vi "Emballage_BDD_codeBarre_bdd.vi"(8 "Error in":errorcluster caption="Error in (no error)") -> (0 "Error out":errorcluster, 3 "tableau ajouté":string[][](array[string]))   [LabVIEW 2020]
uses:
  Modules/FS/60_FS_Controles/60_FS_SetGet.ctl
panel:
  out "tableau_code barre (article)":string[](array[string])
  out "tableau_Produit Code FAS (article)":string[](array[string])
  out "tableau_code barre":string[](array[string])
  out "tableau_Produit Code FAS":string[](array[string])
  out "Result Set":string[][](table) caption="Result Set (from first statement with results)"
  out "Column Names":string[](array[string])
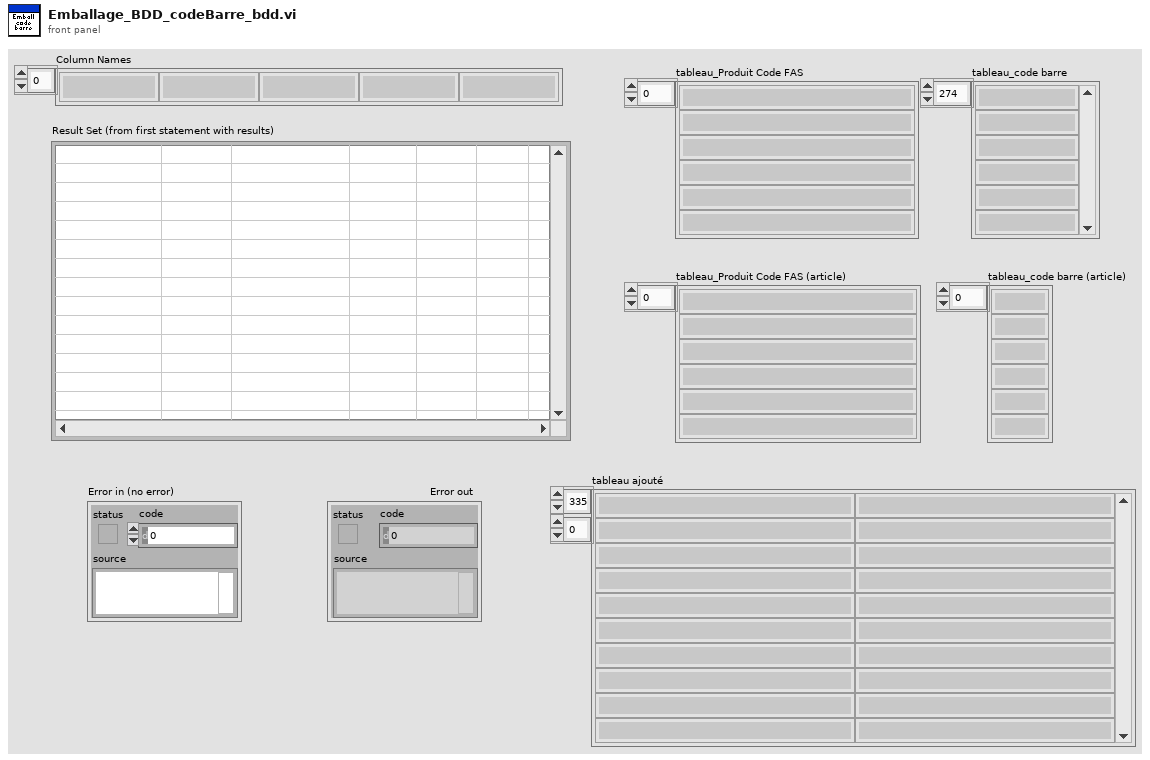
[diagram p1: front panel]
types:
  T1 = typedef "60_FS_SetGet.ctl" = enum16{"set", "get"}
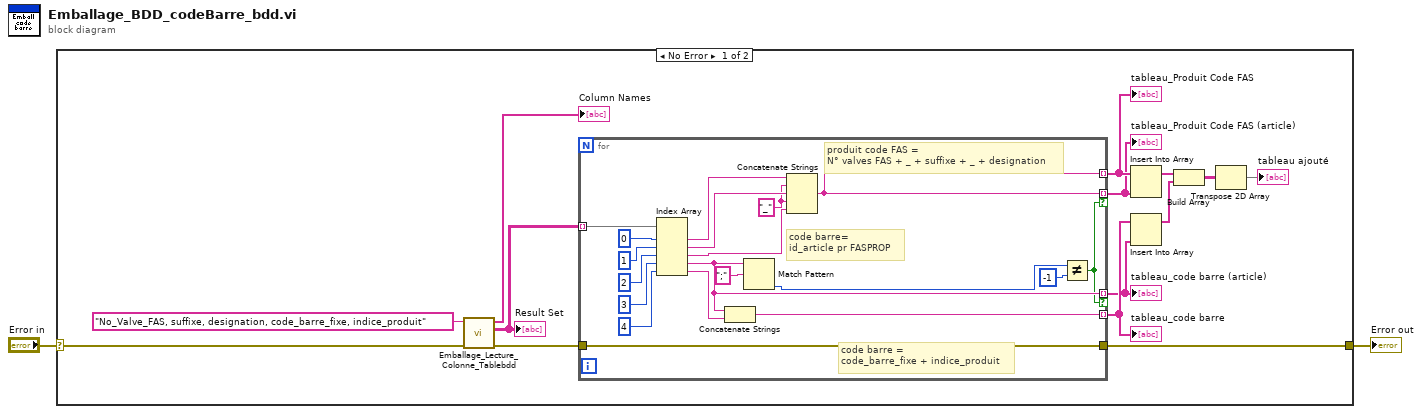
[diagram p0: block diagram]
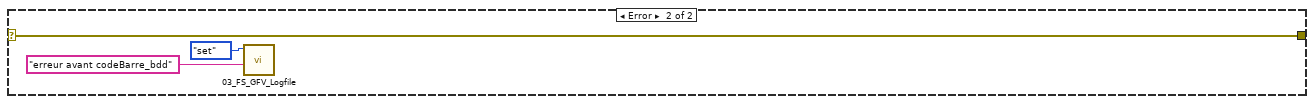
[diagram p2: hidden frame]
diagram:
  n1 = case shown="No Error" "Error in" {
    selector: "Error in" -> [w12 w38]
    tunnel: [w11 w38] -> w1
    frame No Error {
      n2 = call "Emballage_Lecture_Colonne_Tablebdd.vi"("Error in"=w12, "Colonne"="No_Valve_FAS, suffixe, designation, code_barre_fixe, indice_produit") -> ("Error out"=w13:errorcluster, "Result Set"=w14:string[][], "Column Names"=→"Column Names":string[])  [unwired: 6 in, 1 out]
      "Result Set" <- w14
      n3 = for {
        tunnel: w14 -> [w35] mode=indexing
        tunnel: [w19] -> w6 mode=indexing
        tunnel: [w24] -> w4 mode=indexing
        tunnel: w13 -> [w23]
        tunnel: [w23] -> w11
        tunnel: [w19] -> w5 mode=indexing if=w17
        tunnel: [w18] -> w3 mode=indexing if=w17
        w29 = "_" ("chaîne")
        # "code barre=\nid_article pr FASPROP"
        # "code barre =\ncode_barre_fixe + indice_produit"
        # "produit code FAS =\nN° valves FAS + _ + suffixe + _ + designation"
        n4 = Index Array(array=w35, index #1=0 ("indice"), index #2=1 ("indice"), index #3=2 ("indice"), index #4=3 ("indice"), index #5=4 ("indice")) -> (element #1=w31:string, element #2=w30:string, element #3=w28:string, element #4=w18:string, element #5=w25:string)
        n5 = Concatenate Strings(w18, w25) -> (w24:string)
        n6 = Match Pattern(string=w18, regular expression=";" ("expression régulière")) -> (offset past match=w21:i32)  [unwired: 1 in, 3 out]
        n7 = Concatenate Strings(w31, w29, w30, w29, w28) -> (w19:string)
        n8 = Not Equal?(x=w21, y=-1) -> (x != y?=w17:bool)
      }
      "tableau_Produit Code FAS" <- w6
      "tableau_code barre" <- w4
      "tableau_Produit Code FAS (article)" <- w5
      "tableau_code barre (article)" <- w3
      n9 = Insert Into Array(array=w6, new element=w5) -> (w9:string[])  [unwired: 1 in]
      n10 = Insert Into Array(array=w4, new element=w3) -> (w8:string[])  [unwired: 1 in]
      n11 = Build Array(w9, w8) -> (w10:string[][])
      n12 = Transpose 2D Array(2D array=w10) -> (transposed array=→"tableau ajouté":string[][])
    }
    frame Error {
      n13 = call "03_FS_GFV_Logfile.vi"("Chaîne"="erreur avant codeBarre_bdd", "States"=60_FS_SetGet."set") -> ()  [unwired: 8 in, 2 out]
    }
  }
  "Error out" <- w1
